vi "Create.vi"(8 "error in (no error)":errorcluster) -> (0 "error out":errorcluster, 3 "GW-Stop-Cmd out":refnum<class "GW-Stop-Cmd.lvclass">)   [LabVIEW 2013, in "GW-Stop-Cmd.lvclass"]
uses:
  GW-Stop-Cmd.lvclass
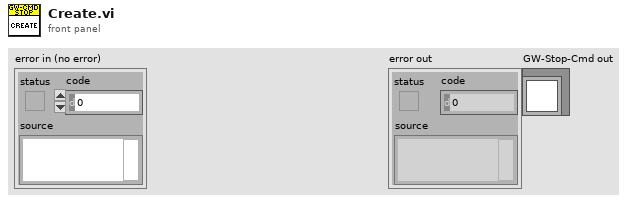
[diagram p1: front panel]
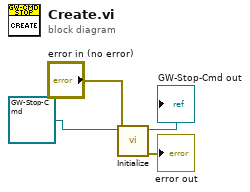
[diagram p0: block diagram]
diagram:
  n1 = call-dynamic "Initialize.vi"("error in (no error)"="error in (no error)", "GW-Stop-Cmd in"=refnum<class "GW-Stop-Cmd.lvclass"> refnum ("GW-Stop-Cmd.lvclass")) -> ("error out"=→"error out":errorcluster, "GW-Stop-Cmd out"=→"GW-Stop-Cmd out":refnum<class "GW-Stop-Cmd.lvclass">)  [unwired: 8 in]
